vi "Steering motor.vi"(8 "Steering position (in pulses)":i64, 9 "Duty Cycle in":sgl, 10 "Switch direction":bool) -> (0 "Duty Cycle out":sgl, 3 "Steering angle(deg)":sgl)   [LabVIEW 2016]
doc: "Inputs\nSteering angle in pulses\nFrequency\nDirection\n'\nThis VI controls the steering motor, via the motor controller. It uses an express VI to send a PWM signal to the motor, with a frequency of 20 000 and a duty cycle which is determined by the control loop. A saftey function is implemented which doesn't allow the motor to go accross +- 45 degrees."
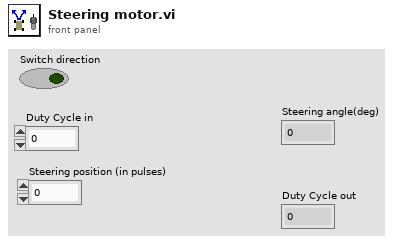
[diagram p1: front panel]
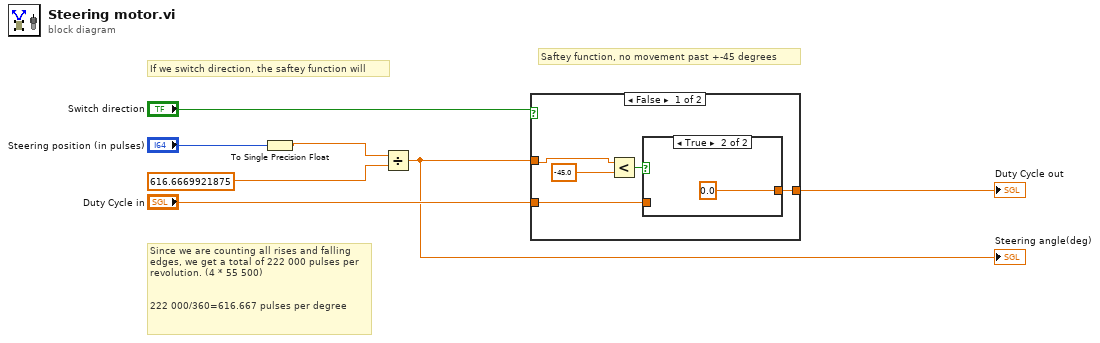
[diagram p0: block diagram]
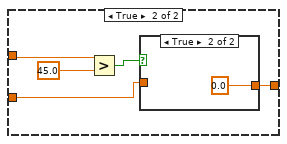
[diagram p3: hidden frame]
diagram:
  # "If we switch direction, the saftey function will"
  # "Since we are counting all rises and falling\nedges, we get a total of 222 000 pulses per\nrevolution. (4 * 55 500)\n \n \n222 000/360=616.667 pulses per degree"
  # "Saftey function, no movement past +-45 degrees"
  n1 = To Single Precision Float(number="Steering position (in pulses)") -> (single precision float=w2:sgl)
  n2 = Divide(x=w2, y=sgl 616.667) -> (x/y=w4:sgl)
  "Steering angle(deg)" <- w4
  n3 = case shown="False" "Switch direction" {
    tunnel: w4 -> [w8 w16]
    tunnel: [w12 w19] -> w1
    tunnel: "Duty Cycle in" -> [w11 w18]
    frame False {
      n4 = Less?(x=w8, y=sgl -45.0) -> (x < y?=w9:bool)
      n5 = case shown="True" w9 {
        tunnel: [w13 sgl 0.0] -> w12
        tunnel: w11 -> [w13 _]
        frame False {
        }
        frame True {
        }
      }
    }
    frame True {
      n6 = Greater?(x=w16, y=sgl 45.0) -> (0:w15:bool)
      n7 = case shown="True" w15 {
        tunnel: [w20 sgl 0.0] -> w19
        tunnel: w18 -> [w20 _]
        frame False {
        }
        frame True {
        }
      }
    }
  }
  "Duty Cycle out" <- w1
